vi "Status Helper.vi"(6 "Number of Data Pts":i32, 7 "Action":T1, 8 "error in (no error)":errorcluster, 11 "Number of Days":i32) -> (0 "error out":errorcluster, 1 "% Push To DB":dbl, 2 "% Get Http Data":dbl, 3 "% Add to QUEUE":dbl, 5 "Number Of Data Points":i32)   [LabVIEW 2012]
uses:
  Status Helper Action.ctl
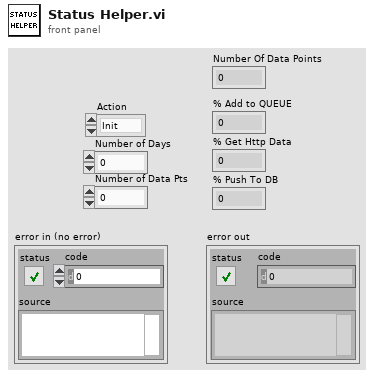
[diagram p1: front panel]
types:
  T1 = typedef "Status Helper Action.ctl" = enum16{"Init", "Load Number Of Days", "Inc Add to Queue ", "Inc Get HTTP Data", "Add Push to DB", "Inc Push To DB", "Read"}
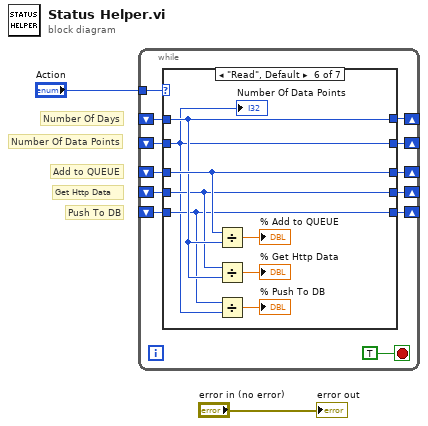
[diagram p0: block diagram]
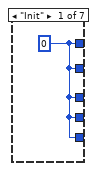
[diagram p2: hidden frame]
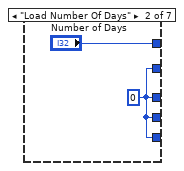
[diagram p3: hidden frame]
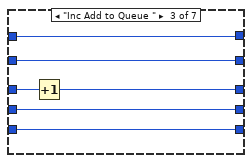
[diagram p4: hidden frame]
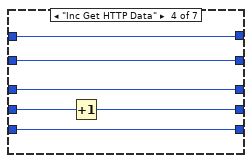
[diagram p5: hidden frame]
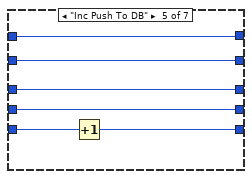
[diagram p6: hidden frame]
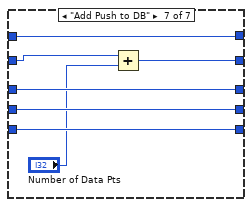
[diagram p7: hidden frame]
diagram:
  # "Number Of Data Points"
  # "Number Of Days"
  # "Push To DB"
  # "Get Http Data"
  # "Add to QUEUE"
  n1 = while {
    tunnel: "Action" -> [w13]
    shift-right: [w10] -> _
    shift-left: _ -> [w7]
    shift-right: [w9] -> _
    shift-left: _ -> [w6]
    shift-right: [w8] -> _
    shift-left: _ -> [w5]
    shift-right: [w12] -> _
    shift-left: _ -> [w11]
    shift-right: [w4] -> _
    shift-left: _ -> [w3]
    stop <- TRUE stop-if-true
    n2 = case shown="\"Read\", Default" w13 {
      tunnel: [w15 "Number of Days" w23 w29 w35 w42 w50] -> w12
      tunnel: w11 -> [_ _ w23 w29 w35 w42 w50]
      tunnel: [w15 w16 w19 w28 w34 w43 w49] -> w10
      tunnel: [w15 w16 w21 w25 w33 w41 w48] -> w9
      tunnel: [w15 w16 w20 w26 w31 w40 w47] -> w8
      tunnel: w7 -> [_ _ w22 w28 w34 w43 w49]
      tunnel: w6 -> [_ _ w21 w27 w33 w41 w48]
      tunnel: w5 -> [_ _ w20 w26 w32 w40 w47]
      tunnel: [w15 w16 w18 w24 w30 w36 w46] -> w4
      tunnel: w3 -> [_ _ w18 w24 w30 w36 w45]
      frame "Init" {
        w15 = 0 ("Number of Days")
      }
      frame "Load Number Of Days" {
        w16 = 0
      }
      frame "Inc Add to Queue " {
        n3 = Increment(x=w22) -> (x+1=w19:i32)
      }
      frame "Inc Get HTTP Data" {
        n4 = Increment(x=w27) -> (x+1=w25:i32)
      }
      frame "Inc Push To DB" {
        n5 = Increment(x=w32) -> (x+1=w31:i32)
      }
      frame "Read", Default {
        n6 = Divide(x=w43, y=w42) -> (x/y=→"% Add to QUEUE":dbl)
        n7 = Divide(x=w41, y=w42) -> (x/y=→"% Get Http Data":dbl)
        n8 = Divide(x=w40, y=w36) -> (x/y=→"% Push To DB":dbl)
        "Number Of Data Points" <- w36
      }
      frame "Add Push to DB" {
        n9 = Add(x=w45, y="Number of Data Pts") -> (x+y=w46:i32)
      }
    }
  }
  "error out" <- "error in (no error)"
